vi "Load Virt Instrs.vi"(8 "error in":errorcluster, 9 "JSON Virt Instrs":T1(array[cluster]), 11 "Host Measure and Stimulus Subsystems in":refnum<class "Host Measure and Stimulus Subsystems.lvclass">) -> (0 "error out":errorcluster, 3 "Host Measure and Stimulus Subsystems out":refnum<class "Host Measure and Stimulus Subsystems.lvclass">)   [LabVIEW 2023, in "HAL GOOP4.lvlib" / "Host Measure and Stimulus Subsystems.lvclass"]
uses:
  Host Measure and Stimulus Subsystems.lvclass
  Host Measure and Stimulus Subsystems.lvclass/Host Measure and Stimulus Subsystems.ctl
  Virtual Instrument Base/Virt Instr Base.lvclass
  <vilib>/Utility/miscctls.llb/LVMapReplaceAction.ctl
  <vilib>/Utility/error.llb/Error Cluster From Error Code.vi
  <vilib>/ErrorRing/Error Ring.xnode
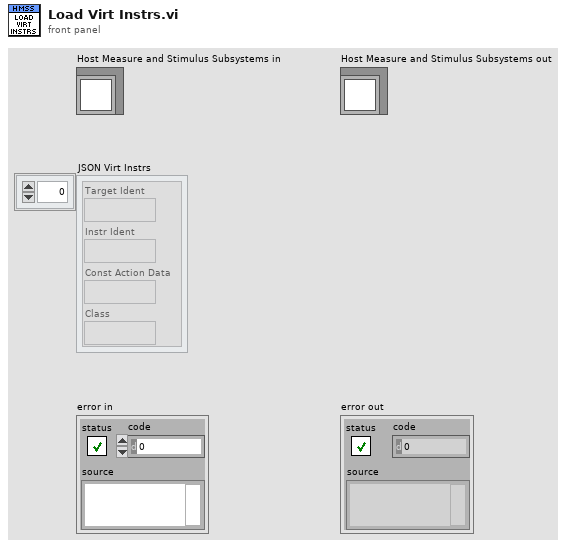
[diagram p1: front panel]
types:
  T1 = cluster{"Target Ident":string, "Instr Ident":string, "Const Action Data":string, "Class":string}[]
  T2 = typedef "LVMapReplaceAction.ctl" = enum32{"Modify Entry only if found", "Add or Modify Entry", "Delete Entry"}
  T3 = map{string, refnum<class "Virt Instr Base.lvclass">}
  T4 = map{string, cluster{"Instrument":refnum<class "Instrument.lvclass">, "Ref Count":u8}}
  T5 = cluster{"Instrument":refnum<class "Instrument.lvclass">, "Ref Count":u8}
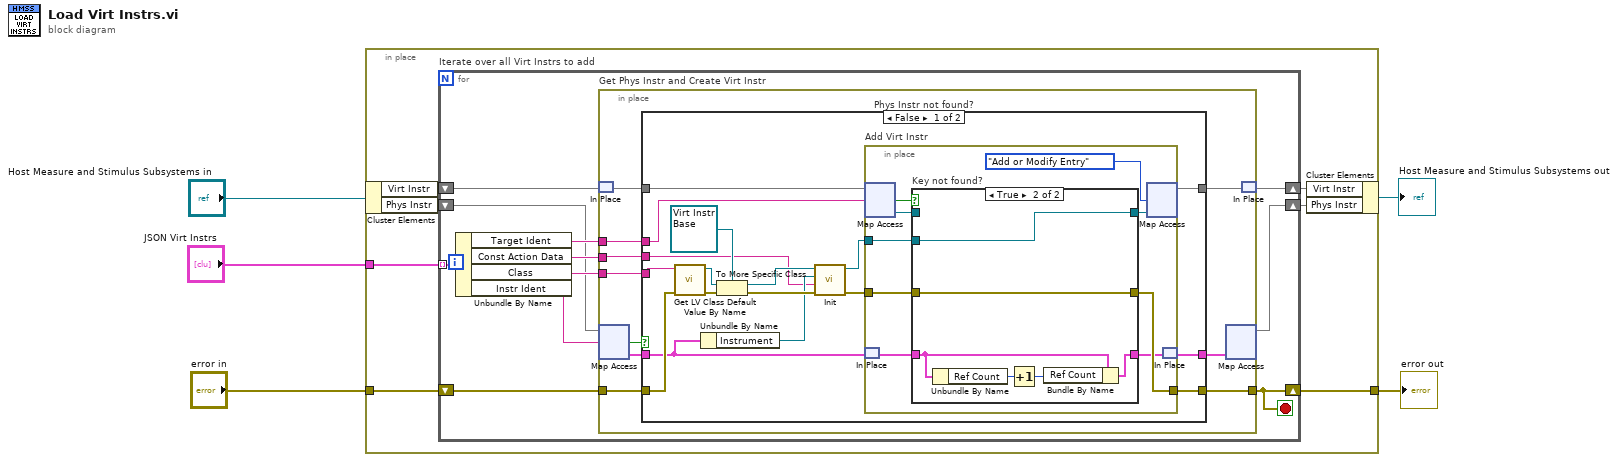
[diagram p0: block diagram]
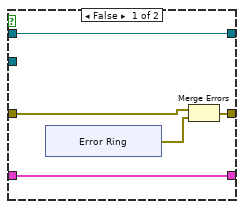
[diagram p2: hidden frame]
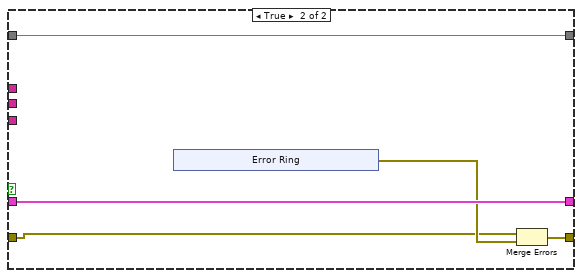
[diagram p3: hidden frame]
diagram:
  n1 = in-place {
    in-place-border: "error in" -> [w12]
    in-place-border: [w11] -> w2
    in-place-border: "JSON Virt Instrs" -> [w10]
    n2 = in-place-cluster #1("Host Measure and Stimulus Subsystems in") -> ("Virt Instr"=w8:T3, "Phys Instr"=w9:T4)
    n3 = for "Iterate over all Virt Instrs to add" {
      tunnel: w10 -> [w23] mode=indexing
      shift-right: [w19] -> w11
      shift-left: w12 -> [w21]
      shift-right: [w14] -> w6
      shift-left: w9 -> [w17]
      shift-right: [w15] -> w7
      shift-left: w8 -> [w16]
      stop <- w19 stop-if-true
      n4 = Unbundle By Name(w23) -> ("Target Ident"=w18:string, "Const Action Data"=w20:string, "Class"=w22:string, "Instr Ident"=w13:string)
      n5 = in-place "Get Phys Instr and Create Virt Instr" {
        in-place-border: w22 -> [w33]
        in-place-border: w21 -> [w32]
        in-place-border: w20 -> [w31]
        in-place-border: [w30] -> w19
        in-place-border: w18 -> [w29]
        n6 = in-place-match #2(w16) -> (w28:T3)
        n7 = in-place-map #3(w17, w13) -> (w26:T5, w24:bool)  [unwired: 1 in]
        n8 = case "Phys Instr not found?" shown="False" w24 {
          tunnel: w33 -> [w50 _]
          tunnel: w32 -> [w49 w76]
          tunnel: w31 -> [w34 _]
          tunnel: [w44 w80] -> w30
          tunnel: w29 -> [w43 _]
          tunnel: w28 -> [w38 w78]
          tunnel: [w37 w78] -> w27
          tunnel: w26 -> [w36 w79]
          tunnel: [w35 w79] -> w25
          frame False {
            n9 = call <vilib>:"Get LV Class Default Value By Name.vi"("error in (no error)"=w49, "class name"=w50) -> ("error out"=w48:errorcluster, "object"=w46:refnum<class>)  [unwired: 8 in]
            n10 = Unbundle By Name(w36) -> ("Instrument"=w39:refnum<class "Instrument.lvclass">)
            n11 = To More Specific Class(target class=refnum<class "Virt Instr Base.lvclass"> refnum ("HAL GOOP4.lvlib:Virtual Instrument Base.lvclass"), reference=w46, error in=w48) -> (specific class reference=w41:refnum<class "Virt Instr Base.lvclass">, error out=w45:errorcluster)
            n12 = call-dynamic "Init.vi"("error in (no error)"=w45, "Constant Action Data"=w34, "HAL GOOP4.lvlib:Instrument"=w39, "Virt Instrument Base in"=w41) -> ("error out"=w42:errorcluster, "Virt Instrument Base out"=w40:refnum<class "Virt Instr Base.lvclass">)  [unwired: 6 in]
            n13 = in-place "Add Virt Instr" {
              in-place-border: w40 -> [w57]
              in-place-border: w42 -> [w55]
              in-place-border: [w54] -> w44
              n14 = in-place-map #4(w38, w43) -> (w58:refnum<class "Virt Instr Base.lvclass">, w59:bool)  [unwired: 1 in]
              n15 = in-place-match #5(w36) -> (w52:T5)
              n16 = case "Key not found?" shown="True" w59 {
                tunnel: w58 -> [w61 _]
                tunnel: w57 -> [_ w70]
                tunnel: [w61 w70] -> w56
                tunnel: w55 -> [w64 w75]
                tunnel: [w62 w75] -> w54
                tunnel: w52 -> [w60 w72]
                tunnel: [w60 w71] -> w51
                frame False {
                  n17 = xnode "Error Ring"() -> ("error out"=w63:errorcluster)
                  n18 = Merge Errors(w64, w63) -> (w62:errorcluster)
                }
                frame True {
                  n19 = Unbundle By Name(w72) -> ("Ref Count"=w74:u8)
                  n20 = Increment(x=w74) -> (x+1=w73:u8)
                  n21 = Bundle By Name(cluster=w72, "Ref Count"=w73) -> (w71:T5)
                }
              }
              n22 = in-place-map #4(w56, LVMapReplaceAction."Add or Modify Entry" ("action")) -> (w37:T3)  [unwired: 2 out]
              n23 = in-place-match #5(w51) -> (w35:T5)
            }
          }
          frame True {
            n24 = xnode "Error Ring"() -> ("error out"=w77:errorcluster)
            n25 = Merge Errors(w76, w77) -> (w80:errorcluster)
          }
        }
        n26 = in-place-map #3(w25) -> (w14:T4)  [unwired: 1 in, 2 out]
        n27 = in-place-match #2(w27) -> (w15:T3)
      }
    }
    n28 = in-place-cluster #1("Virt Instr"=w7, "Phys Instr"=w6) -> (→"Host Measure and Stimulus Subsystems out":refnum<class "Host Measure and Stimulus Subsystems.lvclass">)
  }
  "error out" <- w2
